vi "DiscArchiver.open file.vi"(0 "i ref in":refnum<vi>, 3 "ms timeout (10000)":i32=10000, 5 "error in (no error)":errorcluster) -> (14 "i ref out":refnum<vi>, 17 "timed out":bool, 19 "error out":errorcluster)   [LabVIEW 2014, in "DiscArchiver.lvlib"]
doc: "Opens a new file. The file name is composed by the file prefix plus a number."
uses:
  DiscArchiver.lvlib
  CS_Core/CSSystem/CoreDefs/CoreDefs.error_type.ctl
  CS_Core/CSSystem/CoreLib/CoreLib.lvlib
  CSlibraries-extern/DimLVEvent/LVDimInterface/LVDimInterface.lvlib
  CSlibraries/UtilityLib/UtilityLib.lvlib
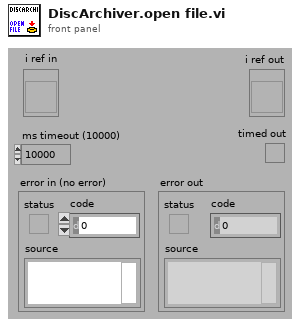
[diagram p1: front panel]
types:
  T1 = typedef "CoreDefs.error_type.ctl" = enum16{"no error", "can't load process", "can't unload process", "process does not exist", "can't install process", "can't remove process", "unknown function", "time out", "can't execute function", "duplicate queue name", "super not found", "caller queue invalid", "can't ping process", "unknown error", "VISA Error", "VISA timeout", "GPIB timeout", "GPIB error", "communication error", "data type mismatch", "can't read data from OPC server", "can't write data to OPC server", "OET error", "function not implemented", "process already exists", "invalid Shared Variable name", "error writing Shared Variable", "error reading Shared Variable", "invalid client name", "corrupt database", "unknown class", "call not authorized", "parameter out of range", "OET timeout: can't get data to modify", "invalid queue name", "requested operation incompatible with current state", "event undefined", "event disabled", "state undefined", "caller is not a friend", "EventBuilder: bad eventID", "EventBuilder: no DAQ devices", "a thread must not stop itself", "UNUSED ELEMENT4", "DiscArchiver: eventData incomplete", "DiscArchiver: eventData does not belong to run", "DiscArchiver: can't open file", "DiscArchiver: can't write to file", "DiscArchiver: available disc space low", "can't acquire semaphore", "error reading data from database", "notifier object is not existing", "can't register process", "can't unregister process", "illegal event type", "object disabled", "object already exists", "can't change state", "Instrument not found", "no connection to remote node", "invalid reference", "N/A", "UNUSED ELEMENT 1", "element not found", "illegal TCP/IP connection detected", "object does not exist", "invalid access ID", "unknown CS system", "invalid privilige", "unsupported data type", "unsupported server type", "IO server already exists", "Shared Variable already exists"}
  T2 = enum16{"open", "open or create", "create or replace", "create", "open (read only)"}
  T3 = typedef "DiscArchiver.lvlib/DiscArchiver.i attribute.ctl" = cluster{"file prefix":string, "actual file":string, "nOfEvents":i32, "file":refnum<file>, "eventBuilder":string, "disc size alarm":bool, "dataDescription":string, "dataDescriptionURL":string, "eventDataURL":string, "headerID":dbl, "completeData":bool, "nOfEventsID":i32, "dataFileID":i32}
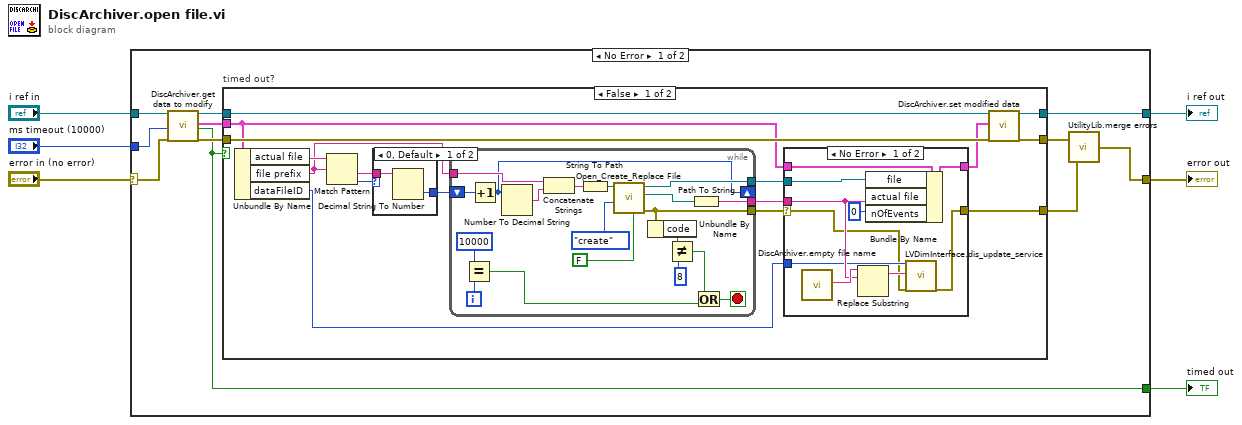
[diagram p0: block diagram]
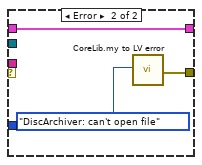
[diagram p2: hidden frame]
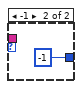
[diagram p3: hidden frame]
diagram:
  n1 = case shown="No Error" "error in (no error)" {
    selector: "error in (no error)" -> [w7 w71]
    tunnel: "i ref in" -> [w17 w72]
    tunnel: [w16 w72] -> w5
    tunnel: "ms timeout (10000)" -> [w12 _]
    tunnel: [w11 _] -> w3
    tunnel: [w8 w71] -> w2
    frame No Error {
      n2 = call "DiscArchiver.get data to modify.vi"("i ref in"=w17, "ms timeout (10000)"=w12, "error in (no error)"=w7) -> ("i ref out"=w15:refnum<vi>, "i attribute"=w13:T3, "timed out"=w11:bool, "error out"=w14:errorcluster)  [unwired: 13 in]
      n3 = case "timed out?" shown="False" w11 {
        tunnel: [w33 w69] -> w10
        tunnel: [w32 w70] -> w16
        tunnel: w15 -> [w31 w70]
        tunnel: w14 -> [w30 w69]
        tunnel: w13 -> [w25 _]
        tunnel: [w21 w69] -> w9
        frame False {
          n4 = Unbundle By Name(w25) -> ("actual file"=w20:string, "file prefix"=w19:string, "dataFileID"=w18:i32)
          n5 = Match Pattern(string=w20, regular expression=w19) -> (after substring=w28:string, offset past match=w29:i32)  [unwired: 1 in, 2 out]
          n6 = case shown="0, Default" w29 {
            tunnel: w28 -> [w67 _]
            tunnel: [w66 -1] -> w27
            frame 0, Default {
              n7 = Decimal String To Number(string=w67) -> (number=w66:i32)  [unwired: 2 in, 1 out]
            }
            frame -1 {
            }
          }
          n8 = while {
            tunnel: w19 -> [w63]
            shift-right: [w50] -> _
            shift-left: w27 -> [w51]
            tunnel: [w58] -> w26
            tunnel: [w48] -> w22
            tunnel: [w57] -> w23
            i -> [w54]
            stop <- w55 stop-if-true
            n9 = Equal?(x=10000, y=w54) -> (x = y?=w52:bool)
            n10 = Increment(x=w51) -> (x+1=w50:i32)
            n11 = Number To Decimal String(number=w50) -> (decimal integer string=w64:string)  [unwired: 1 in]
            n12 = Concatenate Strings(w63, w64) -> (w49:string)
            n13 = String To Path(string=w49) -> (path=w62:path)
            n14 = call <vilib>:"Open_Create_Replace File.vi"("advisory dialog? (display:T)"=FALSE, "function (open:0)"=T2."create", "file path"=w62) -> ("error out"=w58:errorcluster, "new file path"=w47:path, "refnum"=w57:refnum<file>)  [unwired: 5 in, 1 out]
            n15 = Unbundle By Name(w58) -> ("code"=w60:i32)
            n16 = Not Equal?(x=w60, y=8) -> (x != y?=w56:bool)
            n17 = Path To String(path=w47) -> (string=w48:string)
            n18 = Or(x=w56, y=w52) -> (x .or. y?=w55:bool)
          }
          n19 = case shown="No Error" w26 {
            selector: w26 -> [w34 _]
            tunnel: w25 -> [w43 w46]
            tunnel: [w42 w46] -> w24
            tunnel: w23 -> [w41 _]
            tunnel: w22 -> [w36 _]
            tunnel: [w39 w45] -> w21
            tunnel: w18 -> [w35 _]
            frame No Error {
              n20 = call "DiscArchiver.empty file name.vi"() -> ("emptyString"=w37:string)  [unwired: 19 in]
              n21 = Replace Substring(4:w36, 5:w37) -> (1:w38:string)  [unwired: 2 in, 1 out]
              n22 = Bundle By Name(cluster=w43, "file"=w41, "actual file"=w36, "nOfEvents"=0 ("# of items")) -> (w42:T3)
              n23 = call "LVDimInterface.dis_update_service.vi"("my_serviceID"=w35, "data"=w38, "error in (no error)"=w34) -> ("error out"=w39:errorcluster)  [unwired: 14 in, 2 out]
            }
            frame Error {
              n24 = call "CoreLib.my to LV error.vi"("ErrorTypes"=CoreDefs.error_type."DiscArchiver: can't open file") -> ("myErrorCluster"=w45:errorcluster)  [unwired: 17 in, 1 out]
            }
          }
          n25 = call "DiscArchiver.set modified data.vi"("i ref in"=w31, "i attribute"=w24, "error in (no error)"=w30) -> ("i ref out"=w32:refnum<vi>, "error out"=w33:errorcluster)  [unwired: 15 in]
        }
        frame True {
        }
      }
      n26 = call "UtilityLib.merge errors.vi"("error2 (no error)"=w9, "error1 (no error)"=w10) -> ("error out"=w8:errorcluster)
    }
    frame Error {
    }
  }
  "error out" <- w2
  "i ref out" <- w5
  "timed out" <- w3
